vi "ParseTimeStamp.vi"(8 "error in (no error)":errorcluster, 10 "PktData":u8[](array[numeric]) format="%x", 11 "C37.118 PMU in":refnum<class "C37.118 PMU.lvclass">) -> (0 "error out":errorcluster, 1 "Seconds":ext format="%.4f", 2 "PktData":u8[](array[numeric]), 3 "C37.118 PMU out":refnum<class "C37.118 PMU.lvclass">, 4 "TimeQuality":u8, 5 "Stat":u16, 7 "Time Stamp":timestamp)   [LabVIEW 2014, in "SensorPlugins.lvlib" / "C37.118 PMU.lvclass"]
uses:
  C37.118 PMU.lvclass
  C37.118 PMU.lvclass/C37.118 PMU.ctl
  Accessors/Read PMUConfigData.vi
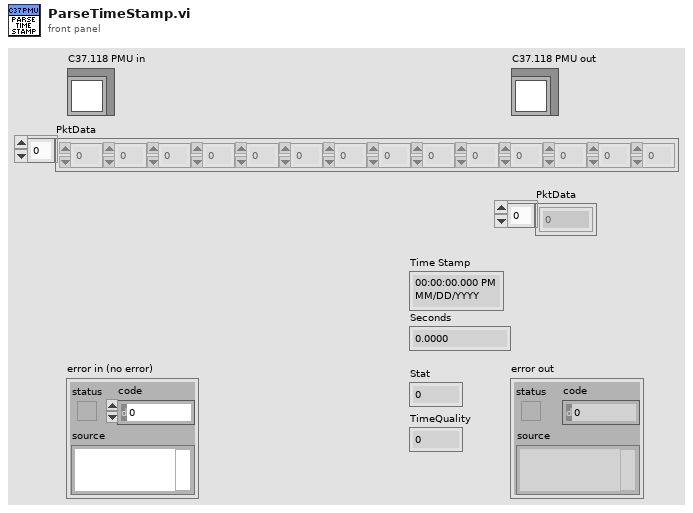
[diagram p1: front panel]
types:
  T1 = typedef "SensorPlugins.lvlib/C37.118 PMU.lvclass/PMUConfigData.ctl" = cluster{"TimeBase":u32, "NUM_PMU":u16, "Station Name":string, "IDCODE":u16, "PHRNMR":u16, "ANNMR":u16, "DIGNMR":u16, "FORMAT BITS":T2, "Valid Inputs":u16[], "DigitalStatusMask":u16[], "24bit_PHUNIT":i32[], "24bit_ANUNIT":u32[], "Analog Amplitude Setting":u32[], "Unit (Vor I)":u8[], "ChannelNames":string, "Fs":i16, "SOC ":u32, "FRACSEC":u32, "F0":sgl, "CFGCNT":u16}
  T2 = typedef "SensorPlugins.lvlib/C37.118 PMU.lvclass/FormatBits.ctl" = cluster{"Rect/Polar":bool, "Phasor Int/Float":bool, "Analog Int/Float":bool, "F/ROCOF Int/Float":bool}
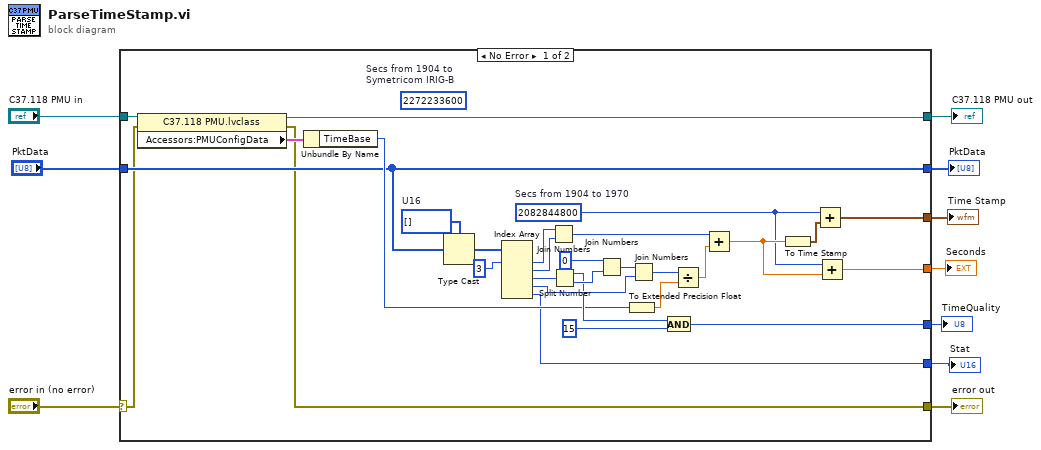
[diagram p0: block diagram]
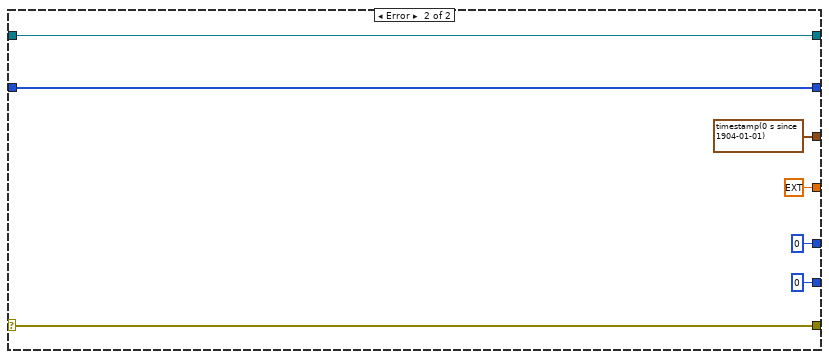
[diagram p2: hidden frame]
diagram:
  n1 = case shown="No Error" "error in (no error)" {
    selector: "error in (no error)" -> [w12 w47]
    tunnel: [w11 w47] -> w9
    tunnel: [w18 w46] -> w7
    tunnel: "C37.118 PMU in" -> [w21 w46]
    tunnel: "PktData" -> [w17 w45]
    tunnel: [w17 w45] -> w5
    tunnel: [w16 timestamp(0 s since 1904-01-01)] -> w4
    tunnel: [w15 ext 0.0] -> w3
    tunnel: [w14 u8 0] -> w2
    tunnel: [w13 u16 0] -> w1
    frame No Error {
      (unwired) u32 2272233600  # Secs from 1904 to Symetricom IRIG-B
      w22 = u32 2082844800  # Secs from 1904 to 1970
      w40 = u16[] []  # U16
      n2 = property class="C37.118 PMU.lvclass"(reference=w21, error in=w12) -> (reference out=w18:refnum<class "C37.118 PMU.lvclass">, error out=w11:errorcluster, "Accessors:PMUConfigData"=w20:T1)
      n3 = Unbundle By Name(w20) -> ("TimeBase"=w19:u32)
      n4 = Type Cast(type=w40, x=w17) -> (*(type *) &x=w39:u16[])
      n5 = Index Array(array=w39, index #1=3 ("index")) -> (element #1=w37:u16, element #2=w36:u16, element #3=w35:u16, element #4=w32:u16, element #5=w13:u16)  [unwired: 4 in]
      n6 = Join Numbers(hi=w37, lo=w36) -> ((hi.lo)=w26:u32)
      n7 = Split Number(x=w35) -> (hi(x)=w28:u8, lo(x)=w34:u8)
      n8 = Join Numbers(hi=u8 0, lo=w34) -> ((hi.lo)=w31:u16)
      n9 = To Extended Precision Float(1:w19) -> (0:w29:ext)
      n10 = Join Numbers(hi=w31, lo=w32) -> ((hi.lo)=w30:u32)
      n11 = And(x=w28, y=u8 15) -> (x .and. y?=w14:u8)
      n12 = Divide(x=w30, y=w29) -> (x/y=w25:ext)
      n13 = Add(x=w26, y=w25) -> (x+y=w23:ext)
      n14 = To Time Stamp(1:w23) -> (0:w24:timestamp)
      n15 = Add(x=w22, y=w24) -> (x+y=w16:timestamp)
      n16 = Add(x=w22, y=w23) -> (x+y=w15:ext)
    }
    frame Error {
    }
  }
  "error out" <- w9
  "C37.118 PMU out" <- w7
  "Time Stamp" <- w4
  "Seconds" <- w3
  "TimeQuality" <- w2
  "Stat" <- w1
  "PktData" <- w5
